vi "display_michelle_visjitter_stopadded_RandCont_PsuedoCO_TSLogFC1.vi"() -> ()   [LabVIEW 2019]
uses:
  <vilib>/Analysis/Matrix/Datatypes/RealMatrix.ctl
  <vilib>/Utility/file.llb/Write Delimited Spreadsheet (DBL).vi
  <vilib>/Analysis/Matrix/NI_Matrix.lvlib
panel:
  out "lambda":dbl
  out "maxITI":dbl
  out "minITI":dbl
  out "goEXP":dbl
  out "meanITI":dbl
  out "Lag1":dbl
  out "TSLog":dbl[][](array[numeric])
  out "TSLog2":dbl[][](array[numeric])
  out "Initialtime":dbl
  out "Time Stamp":timestamp format="%<%H:%M:%S%4u>T"
  out "TSLog1":dbl[][](array[numeric])
  out "ArrayTemp3":T1
  out "StimID2":dbl
  out "Contrast":dbl
  out "TimeOutCounter":i32
  out "ElapsedTime_M":dbl
  out "Base_Contrast":dbl
  out "CurrentTrial":u32=1
  out "Jitter":dbl
  out "BaseITI":dbl
  out "VisStimDuration":dbl
  in  "Stop":bool
  out "Num trials":u32=204
  out "ISI Time":dbl
  out "Stim TS":dbl
  out "Output":dbl[][](array[numeric])
  out "Output frame":T1
  out "Array temp1":T1
  out "Elapsed Time":dbl
  out "Display":bool=TRUE
  out "Trial":u32=1
  out "reward":dbl[](array[numeric])
  out "stim_id":dbl[](array[numeric])
  out "stim_loaded":dbl
  out "Timings":dbl[](array[numeric])
  out "Stimuli Loaded?":bool
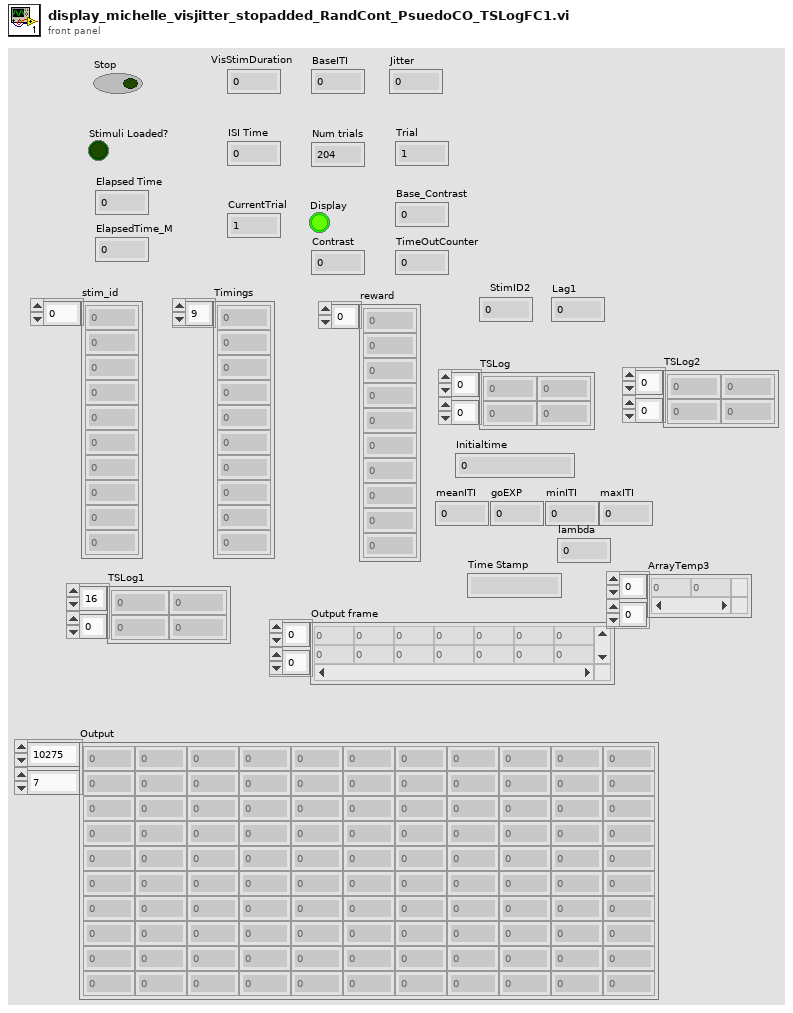
[diagram p1: front panel]
types:
  T1 = typedef "NI_Matrix.lvlib/RealMatrix.ctl" = dbl[][]
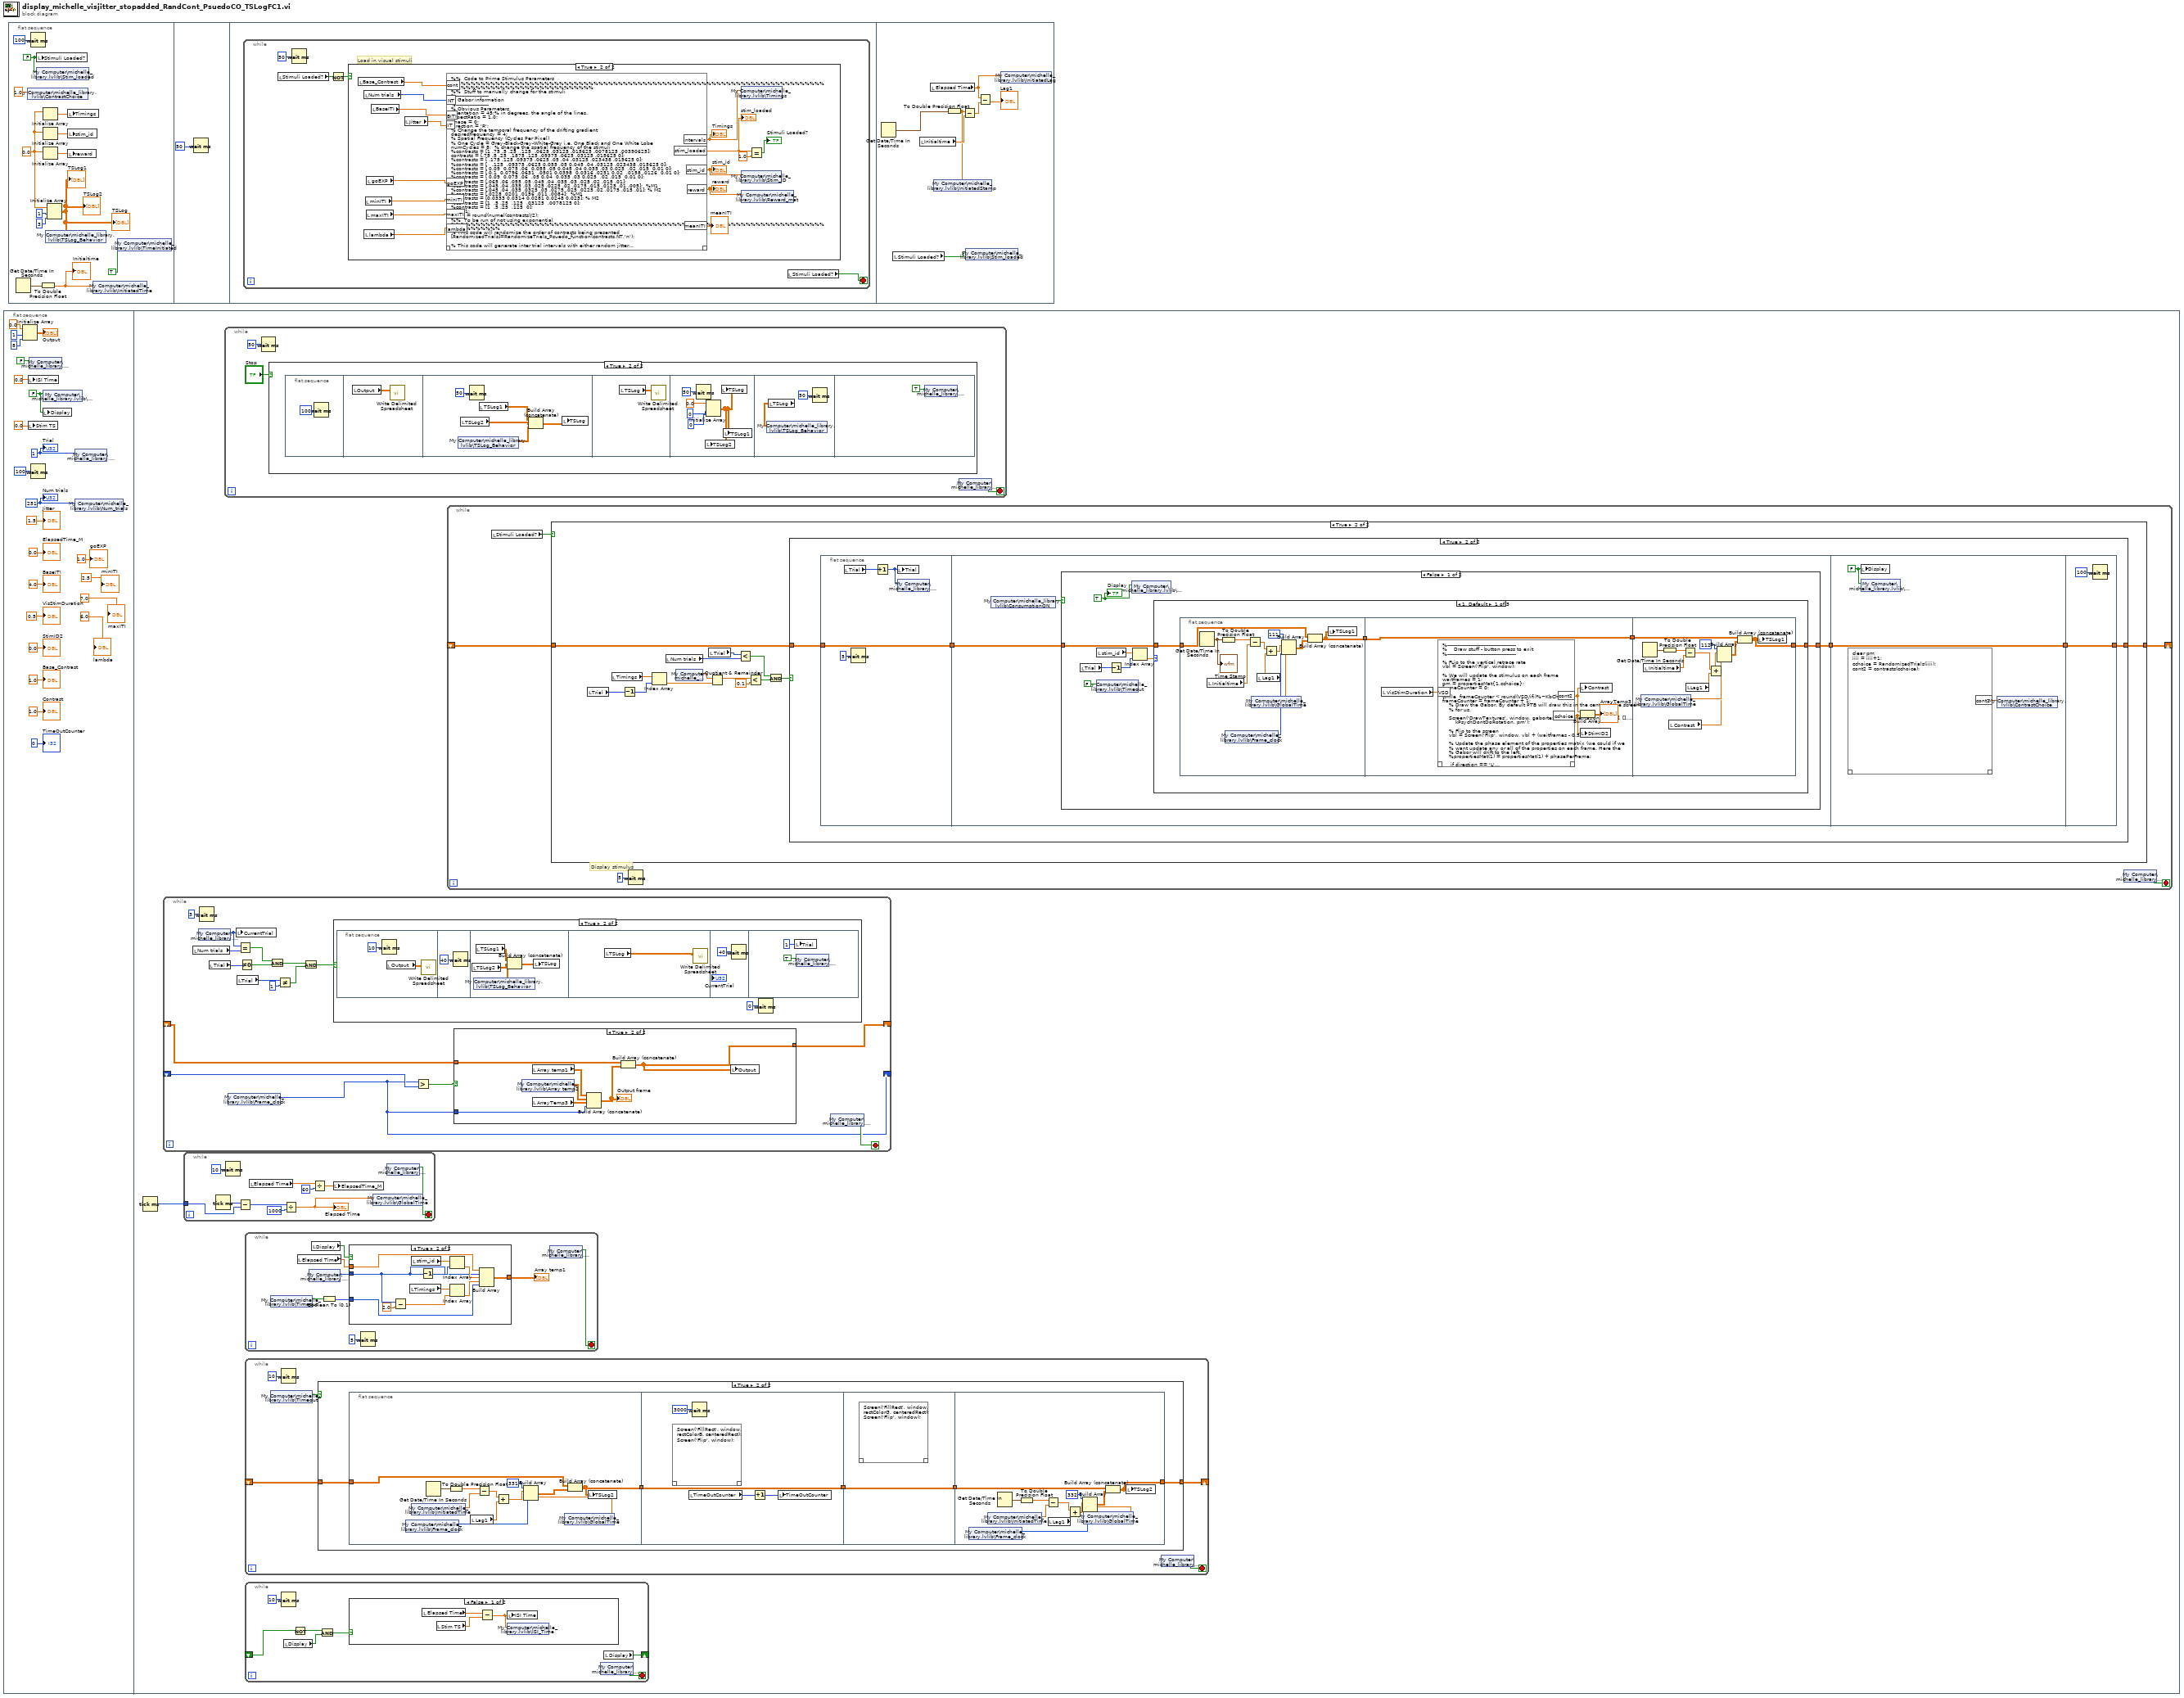
[diagram p0: block diagram]
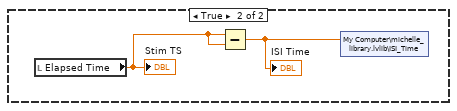
[diagram p5: hidden frame]
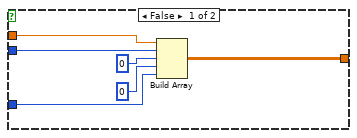
[diagram p6: hidden frame]
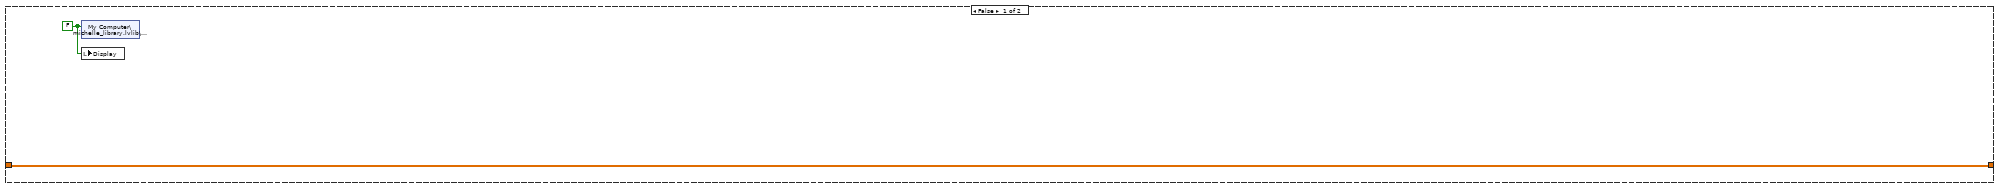
[diagram p10: hidden frame]
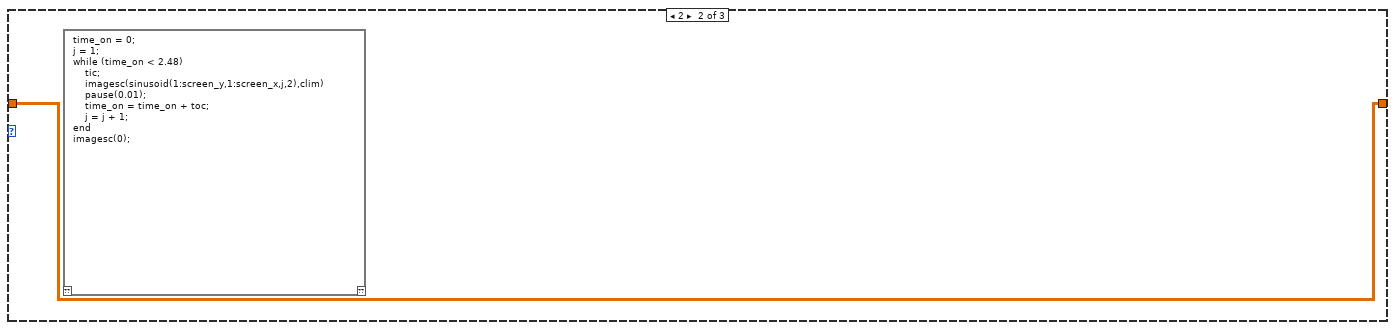
[diagram p11: hidden frame]
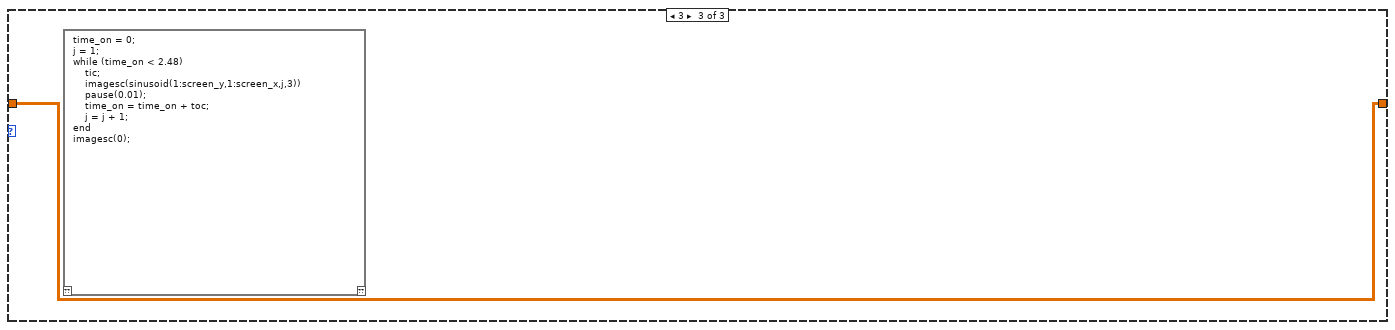
[diagram p12: hidden frame]
diagram:
  n1 = flat-sequence {
    frame #0 {
      w15 = u32 251
      w21 = FALSE ("Display")
      w23 = u32 1 ("Trial")
      n2 = Initialize Array(0.0 ("element"), 1 ("dimension size"), 8 ("dimension size")) -> (→"Output":dbl[][])
      n3 = local write "ISI Time"(0.0 ("ISI Time")) -> ()
      n4 = local write "Stim TS"(0.0 ("Stim TS")) -> ()
      n5 = shared-variable "My Computer\\michelle_library.lvlib\\Stop"(FALSE ("Stop")) -> ()  [unwired: 1 in, 1 out]
      n6 = Wait (ms)(milliseconds to wait=u32 100) -> ()  [unwired: 1 out]
      n7 = shared-variable "My Computer\\michelle_library.lvlib\\Display"(w21) -> ()  [unwired: 1 in, 1 out]
      n8 = local write "Display"(w21) -> ()
      n9 = shared-variable "My Computer\\michelle_library.lvlib\\Trial"(w23) -> ()  [unwired: 1 in, 1 out]
      n10 = shared-variable "My Computer\\michelle_library.lvlib\\Num_trials"(w15) -> ()  [unwired: 1 in, 1 out]
      "Trial" <- w23
      "Num trials" <- w15
      "VisStimDuration" <- 0.5
      "BaseITI" <- 4.0
      "Jitter" <- 1.5
      "Base_Contrast" <- 1.0
      "ElapsedTime_M" <- 0.0
      "TimeOutCounter" <- 0
      "Contrast" <- 1.0
      "StimID2" <- 0.0
      "goEXP" <- 1.0
      "minITI" <- 2.5
      "maxITI" <- 7.0
      "lambda" <- 6.0
    }
    frame #1 {
      n11 = Tick Count (ms)() -> (millisecond timer value=w24:u32)
      n12 = while {
        shift-right: [w134] -> _
        shift-left: _ -> [w135]
        shift-right: [w131] -> _
        shift-left: _ -> [w133]
        stop <- w147 stop-if-true
        n13 = local read "Num trials"() -> (w145:u32)
        n14 = shared-variable "My Computer\\michelle_library.lvlib\\Trial"() -> (w136:u32)  [unwired: 1 in, 1 out]
        n15 = Wait (ms)(milliseconds to wait=u32 3) -> ()  [unwired: 1 out]
        n16 = local read "Trial"() -> (w143:u32)
        n17 = shared-variable "My Computer\\michelle_library.lvlib\\Frame_clock"() -> (w131:u32)  [unwired: 1 in, 1 out]
        n18 = local write "CurrentTrial"(w136) -> ()
        n19 = local read "Trial"() -> (w142:u32)
        n20 = Equal?(x=w136, y=w145) -> (x = y?=w144:bool)
        n21 = Not Equal To 0?(x=w143) -> (x != 0?=w139:bool)
        n22 = And(x=w144, y=w139) -> (x .and. y?=w137:bool)
        n23 = Not Equal?(x=w142, y=1) -> (x != y?=w141:bool)
        n24 = And(x=w137, y=w141) -> (x .and. y?=w138:bool)
        n25 = case shown="True" w138 {
          frame False {
          }
          frame True {
            n26 = flat-sequence {
              frame #0 {
                n27 = Wait (ms)(milliseconds to wait=u32 10) -> ()  [unwired: 1 out]
                n28 = local read "Output"() -> (w158:dbl[][])
                n29 = call-poly <vilib>:"Write Delimited Spreadsheet.vi"("2D data"=w158) -> ()  [unwired: 13 in, 2 out]
              }
              frame #1 {
                n30 = Wait (ms)(milliseconds to wait=u32 40) -> ()  [unwired: 1 out]
              }
              frame #2 {
                n31 = local read "TSLog2"() -> (w163:dbl[][])
                n32 = shared-variable "My Computer\\michelle_library.lvlib\\TSLog_Behavior"() -> (w161:dbl[][])  [unwired: 1 in, 1 out]
                n33 = local read "TSLog1"() -> (w162:dbl[][])
                n34 = Build Array (concatenate) ("Build Matrix")(w162, w163, w161) -> (w160:T1)
                n35 = local write "TSLog"(w160) -> ()
              }
              frame #3 {
                n36 = local read "TSLog"() -> (w164:dbl[][])
                n37 = call-poly <vilib>:"Write Delimited Spreadsheet.vi"("2D data"=w164) -> ()  [unwired: 13 in, 2 out]
              }
              frame #4 {
                n38 = Wait (ms)(milliseconds to wait=u32 40) -> ()  [unwired: 1 out]
              }
              frame #5 {
                n39 = local write "Trial"(1) -> ()
                n40 = shared-variable "My Computer\\michelle_library.lvlib\\Stop"(TRUE) -> ()  [unwired: 1 in, 1 out]
              }
            }
            n41 = Wait (ms)(milliseconds to wait=0) -> ()  [unwired: 1 out]
          }
        }
        n42 = Greater?(x=w131, y=w133) -> (0:w132:bool)
        n43 = case shown="True" w132 {
          tunnel: w135 -> [w148 w151]
          tunnel: [w148 w150] -> w134
          tunnel: w131 -> [_ w149]
          frame False {
          }
          frame True {
            n44 = shared-variable "My Computer\\michelle_library.lvlib\\Array temp2"() -> (w153:dbl[][])  [unwired: 1 in, 1 out]
            n45 = local read "Array temp1"() -> (w152:T1)
            n46 = local read "ArrayTemp3"() -> (w155:T1)
            n47 = Build Array (concatenate)(w152, w153, w155, w149) -> (w154:T1)
            "Output frame" <- w154
            n48 = Build Array (concatenate) ("Build Matrix")(w151, w154) -> (w150:T1)
            n49 = local write "Output"(w150) -> ()
          }
        }
        n50 = shared-variable "My Computer\\michelle_library.lvlib\\Stop"() -> (w147:bool)  [unwired: 1 in, 1 out]
      }
      n51 = while {
        tunnel: w24 -> [w128]
        stop <- w125 stop-if-true
        n52 = Tick Count (ms)() -> (millisecond timer value=w129:u32)
        n53 = Wait (ms)(milliseconds to wait=u32 10) -> ()  [unwired: 1 out]
        n54 = Subtract(x=w129, y=w128) -> (x-y=w126:u32)
        n55 = local read "Elapsed Time"() -> (w123:dbl)
        n56 = Divide(x=w126, y=u32 1000) -> (x/y=w121:dbl)
        "Elapsed Time" <- w121
        n57 = Divide(x=w123, y=60) -> (x/y=w122:dbl)
        n58 = local write "ElapsedTime_M"(w122) -> ()
        n59 = shared-variable "My Computer\\michelle_library.lvlib\\GlobalTime"(w121) -> ()  [unwired: 1 in, 1 out]
        n60 = shared-variable "My Computer\\michelle_library.lvlib\\Stop"() -> (w125:bool)  [unwired: 1 in, 1 out]
      }
      n61 = while {
        stop <- w27 stop-if-true
        n62 = Wait (ms)(milliseconds to wait=50) -> ()  [unwired: 1 out]
        n63 = case shown="True" "Stop" {
          frame False {
          }
          frame True {
            n64 = flat-sequence {
              frame #0 {
                n65 = Wait (ms)(milliseconds to wait=100) -> ()  [unwired: 1 out]
              }
              frame #1 {
                n66 = local read "Output"() -> (w29:dbl[][])
                n67 = call-poly <vilib>:"Write Delimited Spreadsheet.vi"("2D data"=w29) -> ()  [unwired: 13 in, 2 out]
              }
              frame #2 {
                n68 = shared-variable "My Computer\\michelle_library.lvlib\\TSLog_Behavior"() -> (w30:dbl[][])  [unwired: 1 in, 1 out]
                n69 = local read "TSLog2"() -> (w33:dbl[][])
                n70 = Wait (ms)(milliseconds to wait=50) -> ()  [unwired: 1 out]
                n71 = local read "TSLog1"() -> (w32:dbl[][])
                n72 = Build Array (concatenate) ("Build Matrix")(w32, w33, w30) -> (w31:T1)
                n73 = local write "TSLog"(w31) -> ()
              }
              frame #3 {
                n74 = local read "TSLog"() -> (w35:dbl[][])
                n75 = call-poly <vilib>:"Write Delimited Spreadsheet.vi"("2D data"=w35) -> ()  [unwired: 13 in, 2 out]
              }
              frame #4 {
                n76 = Wait (ms)(milliseconds to wait=50) -> ()  [unwired: 1 out]
                n77 = Initialize Array(0.0, 0, 0) -> (w37:dbl[][])
                n78 = local write "TSLog2"(w37) -> ()
                n79 = local write "TSLog"(w37) -> ()
                n80 = local write "TSLog1"(w37) -> ()
              }
              frame #5 {
                n81 = local read "TSLog"() -> (w42:dbl[][])
                n82 = shared-variable "My Computer\\michelle_library.lvlib\\TSLog_Behavior"(w42) -> ()  [unwired: 1 in, 1 out]
                n83 = Wait (ms)(milliseconds to wait=50) -> ()  [unwired: 1 out]
              }
              frame #6 {
                n84 = shared-variable "My Computer\\michelle_library.lvlib\\Stop"(TRUE) -> ()  [unwired: 1 in, 1 out]
              }
            }
          }
        }
        n85 = shared-variable "My Computer\\michelle_library.lvlib\\Stop"() -> (w27:bool)  [unwired: 1 in, 1 out]
      }
      n86 = while {
        stop <- w98 stop-if-true
        n87 = shared-variable "My Computer\\michelle_library.lvlib\\Timeout"() -> (w96:bool)  [unwired: 1 in, 1 out]
        n88 = local read "Elapsed Time"() -> (w102:dbl)
        n89 = shared-variable "My Computer\\michelle_library.lvlib\\Trial"() -> (w100:u32)  [unwired: 1 in, 1 out]
        n90 = local read "Display"() -> (w99:bool)
        n91 = Boolean To (0,1)(Boolean=w96) -> (0, 1=w97:i16)
        n92 = case shown="True" w99 {
          tunnel: w100 -> [w108 w111]
          tunnel: w102 -> [w109 w118]
          tunnel: [w107 w119] -> w101
          tunnel: w97 -> [w104 w113]
          frame False {
            n93 = Build Array(w109, w108, u32 0 ("milliseconds to wait"), 0, w104) -> (w107:T1)
          }
          frame True {
            n94 = Subtract(x=w111, y=2.0) -> (x-y=w110:dbl)
            n95 = local read "Timings"() -> (w116:dbl[])
            n96 = local read "stim_id"() -> (w120:dbl[])
            n97 = Decrement(x=w111) -> (x-1=w115:u32)
            n98 = Index Array(array=w120, index=w115) -> (element=w117:dbl)
            n99 = Index Array(array=w116, index=w110) -> (element=w114:dbl)
            n100 = Build Array(w118, w111, w117, w114, w113) -> (w119:T1)
          }
        }
        "Array temp1" <- w101
        n101 = Wait (ms)(milliseconds to wait=u32 5) -> ()  [unwired: 1 out]
        n102 = shared-variable "My Computer\\michelle_library.lvlib\\Stop"() -> (w98:bool)  [unwired: 1 in, 1 out]
      }
      n103 = while {
        shift-right: [w44] -> _
        shift-left: _ -> [w45]
        stop <- w48 stop-if-true
        n104 = shared-variable "My Computer\\michelle_library.lvlib\\Timeout"() -> (w46:bool)  [unwired: 1 in, 1 out]
        n105 = Wait (ms)(milliseconds to wait=u32 10) -> ()  [unwired: 1 out]
        n106 = case shown="True" w46 {
          tunnel: w45 -> [w49 w54]
          tunnel: [w49 w53] -> w44
          frame False {
          }
          frame True {
            n107 = flat-sequence {
              tunnel: w54 -> [w61]
              tunnel: [w60] -> w51
              tunnel: [w67] -> w52
              tunnel: w51 -> [w67]
              tunnel: w52 -> [w71]
              tunnel: [w71] -> w50
              tunnel: [w77] -> w53
              tunnel: w50 -> [w78]
              frame #0 {
                n108 = shared-variable "My Computer\\michelle_library.lvlib\\Frame_clock"() -> (w55:u32)  [unwired: 1 in, 1 out]
                n109 = shared-variable "My Computer\\michelle_library.lvlib\\InitiatedTime"() -> (w64:dbl)  [unwired: 1 in, 1 out]
                n110 = Get Date/Time In Seconds() -> (seconds since 1Jan1904=w66:timestamp)
                n111 = To Double Precision Float(number=w66) -> (double precision float=w65:dbl)
                n112 = local read "Lag1"() -> (w57:dbl)
                n113 = Subtract(x=w65, y=w64) -> (x-y=w58:dbl)
                n114 = Add(x=w58, y=w57) -> (x+y=w59:dbl)
                n115 = shared-variable "My Computer\\michelle_library.lvlib\\GlobalTime"() -> (w56:dbl)  [unwired: 1 in, 1 out]
                n116 = Build Array(331, w59, w56, w55) -> (w63:T1)
                n117 = Build Array (concatenate) ("Build Matrix")(w61, w63) -> (w60:T1)
                n118 = local write "TSLog2"(w60) -> ()
              }
              frame #1 {
                n119 = script code="Screen('FillRect', window, rectColorB, centeredRect);\nScreen('Flip', window);"() -> ()  [unwired: 1 in, 1 out]
                n120 = local read "TimeOutCounter"() -> (w69:i32)
                n121 = Wait (ms)(milliseconds to wait=u32 3000) -> ()  [unwired: 1 out]
                n122 = Increment(x=w69) -> (x+1=w68:i32)
                n123 = local write "TimeOutCounter"(w68) -> ()
              }
              frame #2 {
                n124 = script code="Screen('FillRect', window, rectColorG, centeredRect);\nScreen('Flip', window);"() -> ()  [unwired: 1 in, 1 out]
              }
              frame #3 {
                n125 = shared-variable "My Computer\\michelle_library.lvlib\\Frame_clock"() -> (w72:u32)  [unwired: 1 in, 1 out]
                n126 = shared-variable "My Computer\\michelle_library.lvlib\\InitiatedTime"() -> (w83:dbl)  [unwired: 1 in, 1 out]
                n127 = Get Date/Time In Seconds() -> (seconds since 1Jan1904=w81:timestamp)
                n128 = To Double Precision Float(number=w81) -> (double precision float=w82:dbl)
                n129 = Subtract(x=w82, y=w83) -> (x-y=w75:dbl)
                n130 = local read "Lag1"() -> (w74:dbl)
                n131 = Add(x=w75, y=w74) -> (x+y=w76:dbl)
                n132 = shared-variable "My Computer\\michelle_library.lvlib\\GlobalTime"() -> (w73:dbl)  [unwired: 1 in, 1 out]
                n133 = Build Array(332, w76, w73, w72) -> (w79:T1)
                n134 = Build Array (concatenate) ("Build Matrix")(w78, w79) -> (w77:T1)
                n135 = local write "TSLog2"(w77) -> ()
              }
            }
          }
        }
        n136 = shared-variable "My Computer\\michelle_library.lvlib\\Stop"() -> (w48:bool)  [unwired: 1 in, 1 out]
      }
      n137 = while {
        shift-right: [w88] -> _
        shift-left: _ -> [w87]
        stop <- w90 stop-if-true
        n138 = Wait (ms)(milliseconds to wait=u32 10) -> ()  [unwired: 1 out]
        n139 = local read "Display"() -> (w85:bool)
        n140 = Not(x=w87) -> (.not. x?=w86:bool)
        n141 = And(x=w86, y=w85) -> (x .and. y?=w84:bool)
        n142 = case shown="False" w84 {
          frame False {
            n143 = local read "Elapsed Time"() -> (w91:dbl)
            n144 = local read "Stim TS"() -> (w93:dbl)
            n145 = Subtract(x=w91, y=w93) -> (x-y=w92:dbl)
            n146 = local write "ISI Time"(w92) -> ()
            n147 = shared-variable "My Computer\\michelle_library.lvlib\\ISI_Time"(w92) -> ()  [unwired: 1 in, 1 out]
          }
          frame True {
            n148 = local read "Elapsed Time"() -> (w94:dbl)
            "Stim TS" <- w94
            n149 = Subtract(x=w94, y=w94) -> (x-y=w95:dbl)
            "ISI Time" <- w95
            n150 = shared-variable "My Computer\\michelle_library.lvlib\\ISI_Time"(w95) -> ()  [unwired: 1 in, 1 out]
          }
        }
        n151 = shared-variable "My Computer\\michelle_library.lvlib\\Stop"() -> (w90:bool)  [unwired: 1 in, 1 out]
        n152 = local read "Display"() -> (w88:bool)
      }
      n153 = while {
        shift-right: [w168] -> _
        shift-left: _ -> [w169]
        stop <- w171 stop-if-true
        # "Display stimulus"
        n154 = local read "Stimuli Loaded?"() -> (w170:bool)
        n155 = case shown="True" w170 {
          tunnel: w169 -> [w173 w175]
          tunnel: [w173 w174] -> w168
          frame False {
          }
          frame True {
            n156 = local read "Trial"() -> (w176:u32)
            n157 = local read "Timings"() -> (w185:dbl[])
            n158 = Decrement(x=w176) -> (x-1=w177:u32)
            n159 = Index Array(array=w185, index=w177) -> (element=w184:dbl)
            n160 = local read "Num trials"() -> (w180:u32)
            n161 = shared-variable "My Computer\\michelle_library.lvlib\\ISI"() -> (w179:dbl)  [unwired: 1 in, 1 out]
            n162 = local read "Trial"() -> (w183:u32)
            n163 = Quotient & Remainder(x=w179, y=w184) -> (x-y*floor(x/y)=w187:dbl)  [unwired: 1 out]
            n164 = Less?(x=w183, y=w180) -> (x < y?=w182:bool)
            n165 = Less?(x=w187, y=0.1) -> (x < y?=w181:bool)
            n166 = And(x=w182, y=w181) -> (x .and. y?=w178:bool)
            n167 = case shown="True" w178 {
              tunnel: w175 -> [w188 w193]
              tunnel: [w188 w192] -> w174
              frame False {
                w189 = FALSE ("Display")
                n168 = shared-variable "My Computer\\michelle_library.lvlib\\Display"(w189) -> ()  [unwired: 1 in, 1 out]
                n169 = local write "Display"(w189) -> ()
              }
              frame True {
                n170 = flat-sequence {
                  tunnel: [w195] -> w194
                  tunnel: w193 -> [w195]
                  tunnel: w194 -> [w200]
                  tunnel: [w199] -> w190
                  tunnel: [w246] -> w191
                  tunnel: w190 -> [w246]
                  tunnel: [w249] -> w192
                  tunnel: w191 -> [w249]
                  frame #0 {
                    n171 = local read "Trial"() -> (w198:u32)
                    n172 = Wait (ms)(milliseconds to wait=u32 5) -> ()  [unwired: 1 out]
                    n173 = Increment(x=w198) -> (x+1=w197:u32)
                    n174 = local write "Trial"(w197) -> ()
                    n175 = shared-variable "My Computer\\michelle_library.lvlib\\Trial"(w197) -> ()  [unwired: 1 in, 1 out]
                  }
                  frame #1 {
                    n176 = shared-variable "My Computer\\michelle_library.lvlib\\ConsumptionON"() -> (w201:bool)  [unwired: 1 in, 1 out]
                    n177 = case shown="False" w201 {
                      tunnel: w200 -> [w203 w245]
                      tunnel: [w202 w245] -> w199
                      frame False {
                        w204 = TRUE ("Boolean")
                        n178 = local read "Trial"() -> (w207:u32)
                        n179 = shared-variable "My Computer\\michelle_library.lvlib\\Timeout"(FALSE) -> ()  [unwired: 1 in, 1 out]
                        n180 = local read "stim_id"() -> (w209:dbl[])
                        n181 = Decrement(x=w207) -> (x-1=w206:u32)
                        n182 = shared-variable "My Computer\\michelle_library.lvlib\\Display"(w204) -> ()  [unwired: 1 in, 1 out]
                        n183 = Index Array(array=w209, index=w206) -> (element=w208:dbl)
                        n184 = case shown="1, Default" w208 {
                          tunnel: w203 -> [w213 w243 w244]
                          tunnel: [w212 w243 w244] -> w202
                          frame 1, Default {
                            n185 = flat-sequence {
                              tunnel: w213 -> [w224]
                              tunnel: [w223] -> w211
                              tunnel: w211 -> [w226]
                              tunnel: [w226] -> w210
                              tunnel: [w241] -> w212
                              tunnel: w210 -> [w240]
                              frame #0 {
                                n186 = Get Date/Time In Seconds() -> (seconds since 1Jan1904=w221:timestamp)
                                "Time Stamp" <- w221
                                n187 = local read "Initialtime"() -> (w219:dbl)
                                n188 = To Double Precision Float(number=w221) -> (double precision float=w220:dbl)
                                n189 = shared-variable "My Computer\\michelle_library.lvlib\\Frame_clock"() -> (w214:u32)  [unwired: 1 in, 1 out]
                                n190 = Subtract(x=w220, y=w219) -> (x-y=w217:dbl)
                                n191 = shared-variable "My Computer\\michelle_library.lvlib\\GlobalTime"() -> (w215:dbl)  [unwired: 1 in, 1 out]
                                n192 = local read "Lag1"() -> (w218:dbl)
                                n193 = Add(x=w217, y=w218) -> (x+y=w216:dbl)
                                n194 = Build Array(111, w216, w215, w214) -> (w222:T1)
                                n195 = Build Array (concatenate) ("Build Matrix")(w224, w222) -> (w223:T1)
                                n196 = local write "TSLog1"(w223) -> ()
                              }
                              frame #1 {
                                n197 = local read "VisStimDuration"() -> (w228:dbl)
                                n198 = script code="%------------------------------------------\n%    Draw stuff - button press to exit\n%------------------------------------------\n\n% FLip to the vertical retrace rate\nvbl = Screen('Flip', window);\n\n% We will update the stimulus on each frame\nwaitframes = 1;\npm = propertiesMat{1,cchoice};\nframeCounter = 0;\ntic\nwhile  frameCounter < round(VSD/ifi)%~KbCheck\nframeCounter = frameCounter + 1;\n    % Draw the Gabor. By default PTB will draw this in the center of the screen\n    % for us.\n   \n    Screen('DrawTextures', window, gabortex, [], [], orientation, [], [], [], [],...\n        kPsychDontDoRotation, pm');\n\n    % Flip to the screen\n    vbl = Screen('Flip', window, vbl + (waitframes - 0.5) * ifi);\n\n    % Update the phase element of the properties matrix (we could if we\n    % want update any or all of the properties on each frame. Here the\n    % Gabor will drift to the left.\n    %propertiesMat(1) = propertiesMat(1) + phasePerFrame;\n \n     if direction == 'L'\n          pm(1) = pm(1) + phasePerFrame;\n     elseif direction =='R'\n          pm(1) = pm(1) - phasePerFrame;\n     end\n\nend\nTime(N) = toc;\nvbl = Screen('Flip', window);"("VSD"=w228) -> ("cont2"=w230:dbl, "cchoice"=w229:dbl)  [unwired: 1 in, 1 out]
                                n199 = local write "Contrast"(w230) -> ()
                                n200 = Build Array(w230, w229) -> (→"ArrayTemp3":T1)
                                n201 = local write "StimID2"(w229) -> ()
                              }
                              frame #2 {
                                n202 = shared-variable "My Computer\\michelle_library.lvlib\\GlobalTime"() -> (w232:dbl)  [unwired: 1 in, 1 out]
                                n203 = Get Date/Time In Seconds() -> (seconds since 1Jan1904=w238:timestamp)
                                n204 = local read "Initialtime"() -> (w237:dbl)
                                n205 = To Double Precision Float(number=w238) -> (double precision float=w236:dbl)
                                n206 = local read "Contrast"() -> (w231:dbl)
                                n207 = Subtract(x=w236, y=w237) -> (x-y=w235:dbl)
                                n208 = local read "Lag1"() -> (w233:dbl)
                                n209 = Add(x=w235, y=w233) -> (x+y=w234:dbl)
                                n210 = Build Array(112, w234, w232, w231) -> (w242:T1)
                                n211 = Build Array (concatenate) ("Build Matrix")(w240, w242) -> (w241:T1)
                                n212 = local write "TSLog1"(w241) -> ()
                              }
                            }
                          }
                          frame 2 {
                            n213 = script code="time_on = 0;\nj = 1;\nwhile (time_on < 2.48)\n    tic;\n    imagesc(sinusoid(1:screen_y,1:screen_x,j,2),clim)\n    pause(0.01);\n    time_on = time_on + toc;\n    j = j + 1;\nend\nimagesc(0);"() -> ()  [unwired: 1 in, 1 out]
                          }
                          frame 3 {
                            n214 = script code="time_on = 0;\nj = 1;\nwhile (time_on < 2.48)\n    tic;\n    imagesc(sinusoid(1:screen_y,1:screen_x,j,3))\n    pause(0.01);\n    time_on = time_on + toc;\n    j = j + 1;\nend\nimagesc(0);"() -> ()  [unwired: 1 in, 1 out]
                          }
                        }
                        "Display" <- w204
                      }
                      frame True {
                      }
                    }
                  }
                  frame #2 {
                    w248 = FALSE ("Display")
                    n215 = script code="clear pm\niiii = iiii+1;\ncchoice = RandomizedTrials(iiii);\ncont2 = contrasts(cchoice);"() -> ("cont2"=w247:dbl)  [unwired: 1 in, 1 out]
                    n216 = local write "Display"(w248) -> ()
                    n217 = shared-variable "My Computer\\michelle_library.lvlib\\Display"(w248) -> ()  [unwired: 1 in, 1 out]
                    n218 = shared-variable "My Computer\\michelle_library.lvlib\\ContrastChoice"(w247) -> ()  [unwired: 1 in, 1 out]
                  }
                  frame #3 {
                    n219 = Wait (ms)(milliseconds to wait=u32 100) -> ()  [unwired: 1 out]
                  }
                }
              }
            }
          }
        }
        n220 = Wait (ms)(milliseconds to wait=u32 5) -> ()  [unwired: 1 out]
        n221 = shared-variable "My Computer\\michelle_library.lvlib\\Stop"() -> (w171:bool)  [unwired: 1 in, 1 out]
      }
    }
  }
  n222 = flat-sequence {
    frame #0 {
      w257 = 0.0 ("element")
      w259 = FALSE ("Stimuli Loaded?")
      n223 = Get Date/Time In Seconds() -> (seconds since 1Jan1904=w254:timestamp)
      n224 = shared-variable "My Computer\\michelle_library.lvlib\\ContrastChoice"(1.0) -> ()  [unwired: 1 in, 1 out]
      n225 = Wait (ms)(milliseconds to wait=u32 100) -> ()  [unwired: 1 out]
      n226 = local write "Stimuli Loaded?"(w259) -> ()
      n227 = shared-variable "My Computer\\michelle_library.lvlib\\Stim_loaded"(w259) -> ()  [unwired: 1 in, 1 out]
      n228 = To Double Precision Float(number=w254) -> (double precision float=w253:dbl)
      "Initialtime" <- w253
      n229 = Initialize Array(w257) -> (w262:dbl[])  [unwired: 1 in]
      n230 = Initialize Array(w257) -> (w261:dbl[])  [unwired: 1 in]
      n231 = Initialize Array(w257) -> (w260:dbl[])  [unwired: 1 in]
      n232 = Initialize Array(w257, 1, 3) -> (w251:dbl[][])
      "TSLog1" <- w251
      "TSLog2" <- w251
      "TSLog" <- w251
      n233 = shared-variable "My Computer\\michelle_library.lvlib\\TSLog_Behavior"(w251) -> ()  [unwired: 1 in, 1 out]
      n234 = local write "Timings"(w262) -> ()
      n235 = local write "stim_id"(w261) -> ()
      n236 = local write "reward"(w260) -> ()
      n237 = shared-variable "My Computer\\michelle_library.lvlib\\InitiatedTime"(w253) -> ()  [unwired: 1 in, 1 out]
      n238 = shared-variable "My Computer\\michelle_library.lvlib\\TimeInitiated"(TRUE) -> ()  [unwired: 1 in, 1 out]
    }
    frame #1 {
      n239 = Wait (ms)(milliseconds to wait=u32 50) -> ()  [unwired: 1 out]
    }
    frame #2 {
      n240 = while {
        stop <- w265 stop-if-true
        # "Load in visual stimuli"
        n241 = local read "Stimuli Loaded?"() -> (w267:bool)
        n242 = Wait (ms)(milliseconds to wait=u32 50) -> ()  [unwired: 1 out]
        n243 = Not(x=w267) -> (.not. x?=w266:bool)
        n244 = case shown="True" w266 {
          frame False {
          }
          frame True {
            n245 = local read "Base_Contrast"() -> (w275:dbl)
            n246 = local read "Num trials"() -> (w278:u32)
            n247 = local read "lambda"() -> (w269:dbl)
            n248 = local read "minITI"() -> (w271:dbl)
            n249 = local read "maxITI"() -> (w270:dbl)
            n250 = local read "goEXP"() -> (w272:dbl)
            n251 = local read "BaseITI"() -> (w277:dbl)
            n252 = local read "Jitter"() -> (w276:dbl)
            n253 = script code="%%  Code to Prime Stimulus Parameters\n%%%%%%%%%%%%%%%%%%%%%%%%%%%%%%%%%%%%%%%%%%%%%%%%%%%%%%%%%%%%%%%%%%%%%%%%%%%%%%%%%%%%%%%%%%%%%%%%%%%%%%%%%\n%%  Stuff to manually change for the stimuli\n%--------------------\n% Gabor information\n%--------------------\n% Obvious Parameters\norientation = 45;% in degrees, the angle of the lines.\naspectRatio = 1.0;\nphase = 0;\ndirection = 'R';\n% Change the temporal frequency of the drifting gradient\ndesiredfrequency = 4;\n% Spatial Frequency (Cycles Per Pixel)\n% One Cycle = Grey-Black-Grey-White-Grey i.e. One Black and One White Lobe\nnumCycles = 8;  % change the spatial frequency of the stimuli\n%contrasts = [1 .75 .5 .25  .125  .0625 .03125 .015625 .0078125 .00390625];\ncontrasts = [.75 .5 .25  .1875 .125 .09375 .0625 .03125 .015625 0];\n%contrasts = [ .175 .125 .09375 .0625 .05 .04 .03125 .023438 .015625 0];\n%contrasts = [   .125  .09375 .0625 0.055 .05 0.045 .04 .03125 .023438 .015625 0];\n%contrasts = [ 0.09  0.075 .06  0.055 .05 0.045 .04 0.035 .03 0.025  .02 .015  0.01 0];\n%contrasts = [ 0.1  0.0796 .0631  .0501 0.0398  0.0316 .0251 0.02  .0158 .0126  0.01 0];\n%contrasts = [ 0.09  0.075 .06  .05 0.04  0.035 .03 0.025  .02 .015  0.01 0];\n%contrasts = [.065 .06 .055 .05 .045 .04 .035 .03 .025 .02 .015 .01];\n%contrasts = [.045 .04 .035 .03 .025 .0225 .02 .0175 .015 .0125 .01 .005];  %M1\n%contrasts = [.045 .04 .035 .0325 .03 .0275 .025 .0225 .02 .0175 .015 .01]; % M2\n%contrasts = [.0228 .0201 .0156 .011 .0084];  %M1\n%contrasts = [0.0333 0.0314 0.0281 0.0248 0.023]; % M2\n%contrasts = [1  .5 .25  .125  .03125  .0078125 0];\n%contrasts = [1  .5 .25  .125  0];\ngo = 1;\nmaxc = round(numel(contrasts)/2);\n%%  To be run of not using exponential\n%%%%%%%%%%%%%%%%%%%%%%%%%%%%%%%%%%%%%%%%%%%%%%%%%%%%%%%%%%%%%%%%%%%%%%%%%%%%%%%%%%%%%%\n% This code will randomize the order of contrasts being presented\n[RandomizedTrials]=RandomizeTrials_Psuedo_function(contrasts,NT,'n');\n\n% This code will generate inter trial intervals with either random jitter\n% or based on an exponential distribution\nif goEXP < 1\n     jit = JIT;\n     jitter = rand(1,NT);\n     jitter = 2*jit*(jitter- .5);\n     ITIbase = BITI;\n     intervals = [ones(1,NT)*ITIbase];\n     intervals = intervals + jitter;\nelseif goEXP > 0\n     intervals = exponentialITI(1/lambda, minITI, maxITI, NT);\nend\n\n%%  Prep the stimulus presentation software\n%%%%%%%%%%%%%%%%%%%%%%%%%%%%%%%%%%%%%%%%%%%%%%%%%%%%%%%%%%%%%%%%%%%%%%%%%%%\nsca;\nclose all;\n% Setup PTB with some default values\nPsychDefaultSetup(2);\n% Set the screen number to the external secondary monitor if there is one connected\nscreenNumber = max(Screen('Screens'));\n\n% Define black, white and grey\nwhite = WhiteIndex(screenNumber);\nblack = BlackIndex(screenNumber);\ngrey = white / 2;\n\n% Open the screen & define it's dimensions\n[window, windowRect] = PsychImaging('OpenWindow', screenNumber, grey,...\n    [], 32, 2, [], [], kPsychNeedRetinaResolution);\n[screenXpixels, screenYpixels] = Screen('WindowSize', window);\n[xCenter, yCenter] = RectCenter(windowRect);\n\n% Get the vertical refresh rate of the monitor\nifi = Screen('GetFlipInterval', window);\n\n% Set maximum priority level\ntopPriorityLevel = MaxPriority(window);\nPriority(topPriorityLevel);\n\n\n% Build a procedural gabor texture (Note: to get a \"standard\" Gabor patch\n% we set a grey background offset, disable normalisation, and set a\n% pre-contrast multiplier of 0.5).\n% Dimension of the region where will draw the Gabor in pixels\ngaborDimPix = windowRect(3);\n% Sigma of Gaussian  (how much to fade around the edges)\nsigma = gaborDimPix / 0;  % change the 0 value to alter the fading\nphasePerFrame = desiredfrequency*360*ifi;\nfreq = numCycles / gaborDimPix;\n\nbackgroundOffset = [0.5 0.5 0.5 0.0];\ndisableNorm = 1;\npreContrastMultiplier = 0.5;\ngabortex = CreateProceduralGabor(window, gaborDimPix, gaborDimPix, [],...\n    backgroundOffset, disableNorm, preContrastMultiplier);\n\n% Randomise the phase of the Gabors and make a properties matrix.\nfor N = 1:numel(contrasts)\npropertiesMat{1,N} = [phase, freq, sigma, contrasts(N), aspectRatio, 0, 0, 0];\nend\n\niiii = 1;\ncchoice = RandomizedTrials(iiii);\ncont2 = contrasts(cchoice);\npm = propertiesMat{1,1};\n\n\n%%  Build up the rectangles for the pause and hold screen\nbaseRect = [0 0 screenXpixels screenYpixels];\ncenteredRect = CenterRectOnPointd(baseRect, xCenter, yCenter);\nrectColorB = [0 0 0];\nrectColorG = [128 128 128]/255;\n\n%%  Finalize the trial data and orders\nstim_id = [ones(1,NT)*1];\nreward = [ones(1,NT)*1];\nmeanITI = nanmean(intervals);\nrand_idx1 = randperm(NT);\nrand_idx2 = randperm(NT);\nintervals = intervals(rand_idx2);\nstim_id = stim_id(rand_idx2);\nreward = reward(rand_idx2);\n%%  All Done!\n%  indicate that the necessary preloading of data has been completed.\nstim_loaded = 1;" ("Script Node")("NT"=w278, "BITI"=w277, "JIT"=w276, "cont"=w275, "goEXP"=w272, "minITI"=w271, "maxITI"=w270, "lambda"=w269) -> ("stim_loaded"=w283:dbl, "intervals"=w279:dbl[], "stim_id"=w280:dbl[], "reward"=w281:dbl[], "meanITI"=→"meanITI":dbl)  [unwired: 1 in, 1 out]
            "stim_loaded" <- w283
            "Timings" <- w279
            "stim_id" <- w280
            "reward" <- w281
            n254 = shared-variable "My Computer\\michelle_library.lvlib\\Timings"(w279) -> ()  [unwired: 1 in, 1 out]
            n255 = shared-variable "My Computer\\michelle_library.lvlib\\Stim_ID"(w280) -> ()  [unwired: 1 in, 1 out]
            n256 = shared-variable "My Computer\\michelle_library.lvlib\\Reward_mat"(w281) -> ()  [unwired: 1 in, 1 out]
            n257 = Equal?(x=w283, y=1.0) -> (x = y?=→"Stimuli Loaded?":bool)
          }
        }
        n258 = local read "Stimuli Loaded?"() -> (w265:bool)
      }
    }
    frame #3 {
      n259 = Get Date/Time In Seconds() -> (seconds since 1Jan1904=w290:timestamp)
      n260 = local read "Stimuli Loaded?"() -> (w285:bool)
      n261 = local read "Initialtime"() -> (w289:dbl)
      n262 = local read "Elapsed Time"() -> (w284:dbl)
      n263 = To Double Precision Float(number=w290) -> (double precision float=w287:dbl)
      n264 = shared-variable "My Computer\\michelle_library.lvlib\\InitiatedStamp"(w287) -> ()  [unwired: 1 in, 1 out]
      n265 = Subtract(x=w287, y=w289) -> (x-y=w288:dbl)
      n266 = shared-variable "My Computer\\michelle_library.lvlib\\Stim_loaded"(w285) -> ()  [unwired: 1 in, 1 out]
      n267 = Subtract(x=w284, y=w288) -> (x-y=→"Lag1":dbl)
      n268 = shared-variable "My Computer\\michelle_library.lvlib\\InitiatedLag"(w284) -> ()  [unwired: 1 in, 1 out]
    }
  }
